vi "OC_Branch_core.vi"(9 "if set/clear":bool, 10 "flag":enum8{"C", "Z", "I", "D", "B", "V", "N"}(ring)=enum."Z", 11 "registers":T1={"A"=0, "X"=0, "Y"=0, "SP"=253, "PC"=0, "P"=36} {"P" format="%08b"; "PC" format="%04x"; "SP" format="%02x"; "Y" format="%02x"; "X" format="%02x"; "A" format="%02x"}) -> (3 "registers":T1 {"P" format="%08b"; "PC" format="%04x"; "SP" format="%02x"; "Y" format="%02x"; "X" format="%02x"; "A" format="%02x"})   [LabVIEW 2018]
uses:
  CPU_registers.ctl
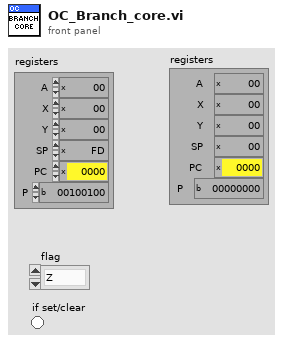
[diagram p1: front panel]
types:
  T1 = typedef "CPU_registers.ctl" = cluster{"A":u8, "X":u8, "Y":u8, "SP":u8, "PC":u16, "P":u8}
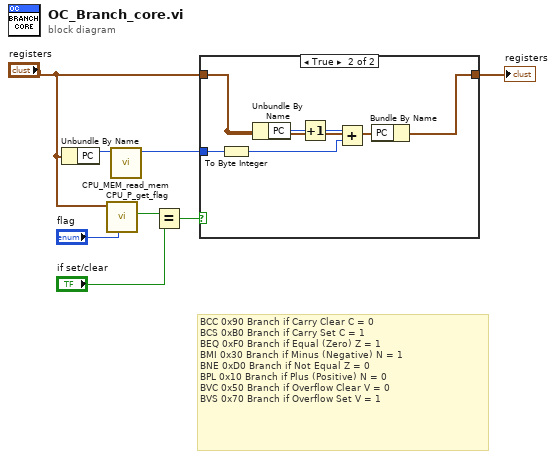
[diagram p0: block diagram]
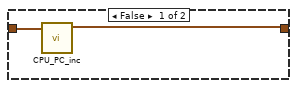
[diagram p2: hidden frame]
diagram:
  # "BCC\t0x90\tBranch if Carry Clear\tC = 0\nBCS\t0xB0\tBranch if Carry Set\tC = 1\nBEQ\t0xF0\tBranch if Equal (Zero)\tZ = 1\nBMI\t0x30\tBranch if Minus (Negative)\tN = 1\nBNE\t0xD0\tBranch if Not Equal\tZ = 0\nBPL\t0x10\tBranch if Plus (Positive)\tN = 0\nBVC\t0x50\tBranch if Overflow Clear\tV = 0\nBVS\t0x70\tBranch if Overflow Set\tV = 1"
  n1 = Unbundle By Name("registers") -> ("PC"=w8:u16)
  n2 = call "CPU_P_get_flag.vi"("flag"="flag", "registers"="registers") -> ("Value"=w5:bool)  [unwired: 8 in, 1 out]
  n3 = call "CPU_MEM_read_mem.vi"("address"=w8) -> ("value out"=w2:u8)  [unwired: 10 in]
  n4 = Equal?(x=w5, y="if set/clear") -> (x = y?=w4:bool)
  n5 = case shown="True" w4 {
    tunnel: "registers" -> [w10 w17]
    tunnel: [w9 w16] -> w6
    tunnel: w2 -> [_ w13]
    frame False {
      n6 = call "CPU_PC_inc.vi"("registers"=w10) -> ("registers"=w9:T1)  [unwired: 10 in]
    }
    frame True {
      n7 = To Byte Integer(number=w13) -> (8bit integer=w12:i8)
      n8 = Unbundle By Name(w17) -> ("PC"=w15:u16)
      n9 = Increment(x=w15) -> (x+1=w11:u16)
      n10 = Add(x=w11, y=w12) -> (x+y=w14:u16)
      n11 = Bundle By Name(cluster=w17, "PC"=w14) -> (w16:T1)
    }
  }
  "registers" <- w6
